vi "storage_run.vi"() -> ()   [LabVIEW 2019]
uses:
  lib/libSimulationControl/libSimulationControl.lvlib
  lib/libFileFunctions/libFileFunctions.lvlib
panel:
  out "outputFiles source":path
  out "storage path":path
  out "full_names":string[](array[string])
  # "*******************************************************************\nBiogas Plant Control\n\nAuthor: Paul Zügel\nGCSC-Frankfurt am Main 2020\n\n*******************************************************************"
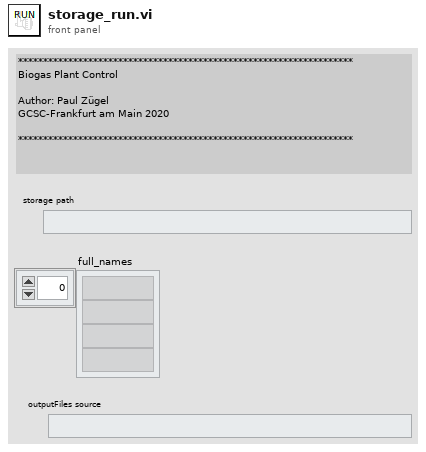
[diagram p1: front panel]
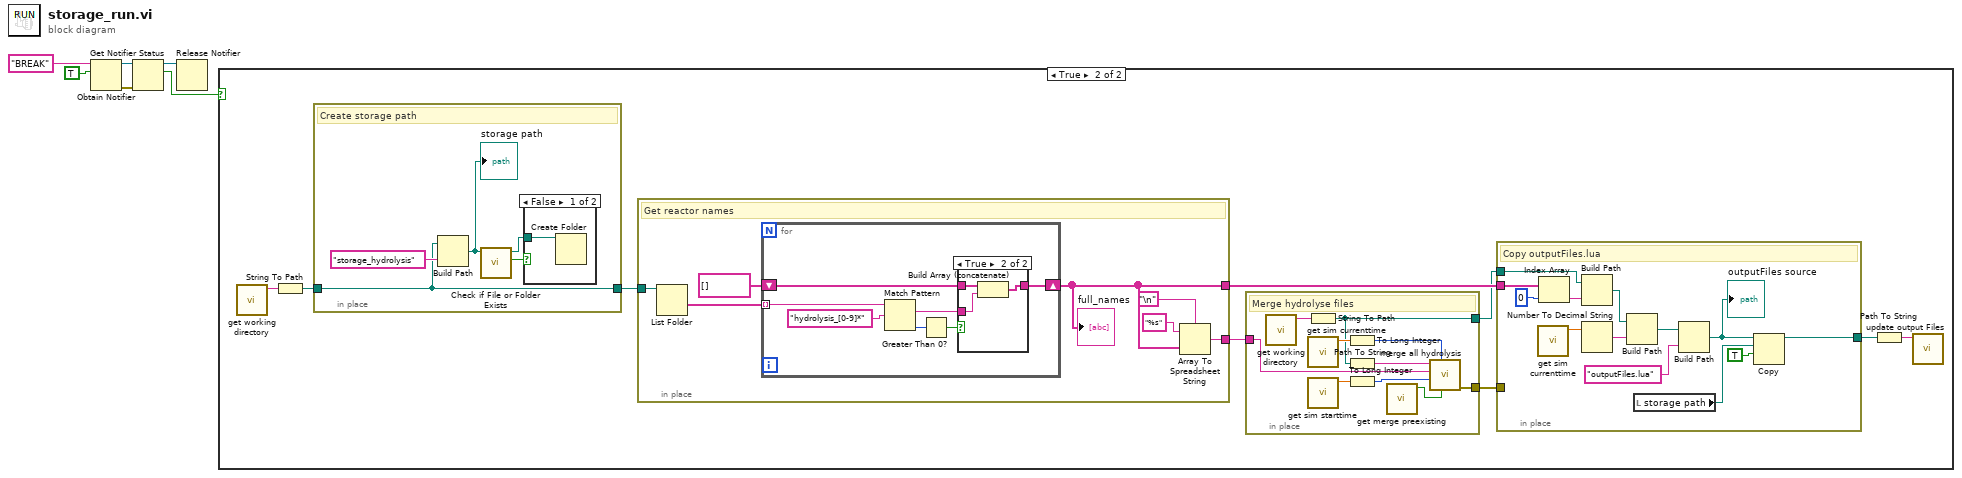
[diagram p0: block diagram]
diagram:
  # "Copy file"
  n1 = Obtain Notifier(name (unnamed)="BREAK", notification data type=TRUE) -> (notifier out=w4:refnum<notifier>, error out=w3:errorcluster)  [unwired: 2 in, 1 out]
  n2 = Get Notifier Status(notifier=w4, error in (no error)=w3) -> (notifier out=w1:refnum<notifier>, current notification=w2:bool)  [unwired: 3 out]
  n3 = Release Notifier(notifier=w1) -> ()  [unwired: 2 in, 3 out]
  n4 = case shown="True" w2 {
    frame False {
    }
    frame True {
      n5 = call "get working directory.vi"() -> ("function return"=w8:string)  [unwired: 10 in, 1 out]
      n6 = String To Path(string=w8) -> (path=w9:path)
      n7 = in-place {
        in-place-border: w9 -> [w16]
        in-place-border: [w16] -> w7
        # "Create storage path"
        n8 = Build Path(base path=w16, name or relative path="storage_hydrolysis") -> (appended path=w19:path)
        "storage path" <- w19
        n9 = call <vilib>:"Check if File or Folder Exists.vi"("path"=w19) -> ("file or folder exists?"=w18:bool, "dup path"=w17:path)  [unwired: 8 in, 1 out]
        n10 = case shown="False" w18 {
          tunnel: w17 -> [w21 _]
          frame False {
            n11 = Create Folder(path (use dialog)=w21) -> ()  [unwired: 2 in, 3 out]
          }
          frame True {
          }
        }
      }
      n12 = in-place {
        in-place-border: w7 -> [w49]
        in-place-border: [w46] -> w15
        in-place-border: [w45] -> w13
        # "Get reactor names"
        n13 = List Folder(path=w49) -> (folder names=w51:string[])  [unwired: 3 in, 3 out]
        n14 = for {
          tunnel: w51 -> [w52] mode=indexing
          shift-right: [w53] -> w45
          shift-left: string[] [] -> [w55]
          n15 = Match Pattern(string=w52, regular expression="hydrolysis_[0-9]*") -> (match substring=w54:string, offset past match=w56:i32)  [unwired: 1 in, 2 out]
          n16 = Greater Than 0?(x=w56) -> (x > 0?=w57:bool)
          n17 = case shown="True" w57 {
            tunnel: [w59 w62] -> w53
            tunnel: w55 -> [w59 w61]
            tunnel: w54 -> [_ w60]
            frame False {
            }
            frame True {
              n18 = Build Array (concatenate)(w61, w60) -> (w62:string[])
            }
          }
        }
        "full_names" <- w45
        n19 = Array To Spreadsheet String(delimiter (Tab)="\n", array=w45, 3:"%s" ("format string")) -> (spreadsheet string=w46:string)
      }
      n20 = in-place {
        in-place-border: w15 -> [w44]
        in-place-border: [w37] -> w14
        in-place-border: [w36] -> w12
        # "Merge hydrolyse files"
        n21 = call "get working directory.vi"() -> ("function return"=w43:string)  [unwired: 10 in, 1 out]
        n22 = String To Path(string=w43) -> (path=w36:path)
        n23 = call "get sim currenttime.vi"() -> ("current_time"=w41:dbl)  [unwired: 10 in, 1 out]
        n24 = call "get sim starttime.vi"() -> ("sim_starttime"=w40:dbl)  [unwired: 10 in, 1 out]
        n25 = To Long Integer(number=w41) -> (32bit integer=w39:i32)
        n26 = Path To String(path=w36) -> (string=w42:string)
        n27 = To Long Integer(number=w40) -> (32bit integer=w38:i32)
        n28 = call "get merge preexisting.vi"() -> ("function return"=w35:bool)  [unwired: 10 in, 1 out]
        n29 = call "merge all hydrolysis.vi"("merge_preexisting"=w35, "current_starttime"=w39, "simulation_starttime"=w38, "reactor_names"=w44, "working_dir"=w42) -> ("error out"=w37:errorcluster)  [unwired: 6 in]
      }
      n30 = in-place {
        in-place-border: w14 -> [_]
        in-place-border: w13 -> [w34]
        in-place-border: w12 -> [w30]
        in-place-border: [w22] -> w11
        # "Copy outputFiles.lua"
        n31 = call "get sim currenttime.vi"() -> ("current_time"=w29:dbl)  [unwired: 10 in, 1 out]
        n32 = Index Array(array=w34, index=0) -> (element=w32:string)
        n33 = Build Path(base path=w30, name or relative path=w32) -> (appended path=w28:path)
        n34 = Number To Decimal String(number=w29) -> (decimal integer string=w27:string)  [unwired: 1 in]
        n35 = Build Path(base path=w28, name or relative path=w27) -> (appended path=w26:path)
        n36 = local read "storage path"() -> (w24:path)
        n37 = Build Path(base path=w26, name or relative path="outputFiles.lua") -> (appended path=w25:path)
        "outputFiles source" <- w25
        n38 = Copy(9:TRUE ("overwrite (F)"), 10:w24, 11:w25) -> (3:w22:path)  [unwired: 2 in, 2 out]
      }
      n39 = Path To String(path=w11) -> (string=w10:string)
      n40 = call "update output Files.vi"("outputFiles_path"=w10) -> ()  [unwired: 10 in, 1 out]
    }
  }
